vi "Configure.vi"(8 "error in (no error)":errorcluster caption="错误输入（无错误）", 11 "5720A 输入":refnum<class "5720A.lvclass">) -> (0 "error out":errorcluster caption="错误输出", 3 "5720A 输出":refnum<class "5720A.lvclass">)   [LabVIEW 2020, in "5720A.lvlib" / "5720A.lvclass"]
uses:
  5720A.lvclass
  <instrlib>/Fluke 5XXX Series Multicalibrators/Fluke 5XXX Series Multicalibrators.lvlib
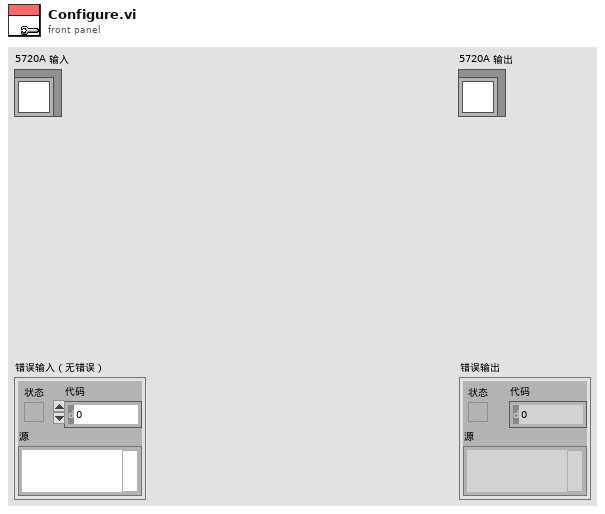
[diagram p1: front panel]
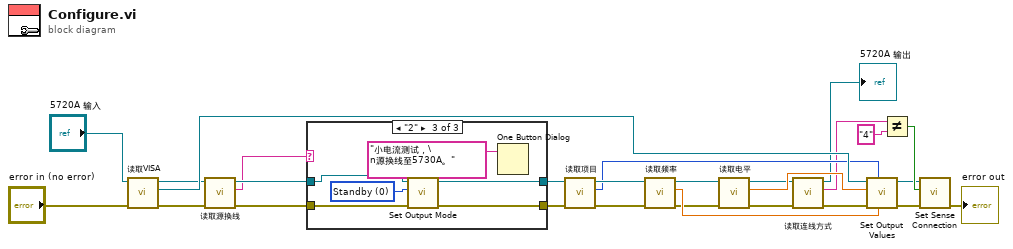
[diagram p0: block diagram]
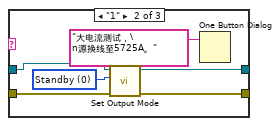
[diagram p3: hidden frame]
diagram:
  n1 = call "读取VISA.vi"("error in (no error)"="error in (no error)", "多功能校准源接口输入"="5720A 输入") -> ("error out"=w6:errorcluster, "VISA"=w26:refnum<visa-resource-name>, "多功能校准源接口输出"=w7:refnum<class "5720A.lvclass">)  [unwired: 7 in]
  n2 = call "读取源换线.vi"("error in (no error)"=w6, "多功能校准源接口输入"=w7) -> ("error out"=w3:errorcluster, "源换线"=w1:string, "多功能校准源接口输出"=w5:refnum<class "5720A.lvclass">)  [unwired: 7 in]
  n3 = case shown="\"2\"" w1 {
    tunnel: w5 -> [w29 w35 w41]
    tunnel: [w29 w32 w38] -> w4
    tunnel: w3 -> [w28 w31 w37]
    tunnel: [w28 w30 w36] -> w2
    frame "0", Default {
    }
    frame "1" {
      w34 = u32 0 items=["Standby", "Operate"] ("Output Mode")
      n4 = call-dynamic "Set Output Mode.vi"("error in (no error)"=w31, "Output Mode"=w34, "5720A 输入"=w35) -> ("error out"=w30:errorcluster, "5720A 输出"=w32:refnum<class "5720A.lvclass">)  [unwired: 7 in]
      n5 = One Button Dialog(message="大电流测试，\n源换线至5725A。" ("消息")) -> ()  [unwired: 1 in, 1 out]
    }
    frame "2" {
      w40 = u32 0 items=["Standby", "Operate"] ("Output Mode")
      n6 = call-dynamic "Set Output Mode.vi"("error in (no error)"=w37, "Output Mode"=w40, "5720A 输入"=w41) -> ("error out"=w36:errorcluster, "5720A 输出"=w38:refnum<class "5720A.lvclass">)  [unwired: 7 in]
      n7 = One Button Dialog(message="小电流测试，\n源换线至5730A。" ("消息")) -> ()  [unwired: 1 in, 1 out]
    }
  }
  n8 = call "读取项目.vi"("error in (no error)"=w2, "多功能校准源接口输入"=w4) -> ("error out"=w22:errorcluster, "项目"=w16:u32, "多功能校准源接口输出"=w19:refnum<class "5720A.lvclass">)  [unwired: 7 in]
  n9 = call "读取频率.vi"("error in (no error)"=w22, "多功能校准源接口输入"=w19) -> ("error out"=w21:errorcluster, "频率"=w25:dbl, "多功能校准源接口输出"=w20:refnum<class "5720A.lvclass">)  [unwired: 7 in]
  n10 = call "读取电平.vi"("error in (no error)"=w21, "多功能校准源接口输入"=w20) -> ("error out"=w14:errorcluster, "电平"=w24:dbl, "多功能校准源接口输出"=w15:refnum<class "5720A.lvclass">)  [unwired: 7 in]
  n11 = call "读取连线方式.vi"("error in (no error)"=w14, "多功能校准源接口输入"=w15) -> ("error out"=w13:errorcluster, "连线方式"=w10:string, "多功能校准源接口输出"=→"5720A 输出":refnum<class "5720A.lvclass">)  [unwired: 7 in]
  n12 = call <instrlib>:"Set Output Values.vi"("Fundamental Frequency (0.0 Hz)"=w25, "Output Value(s) (0 - Amplitude)"=w16, "error in (no error)"=w13, "Primary Value (0.0)"=w24, "VISA resource name"=w26) -> ("error out"=w18:errorcluster, "VISA resource name out"=w8:refnum<visa-resource-name>)  [unwired: 5 in]
  n13 = Not Equal?(x=w10, y="4") -> (x != y?=w9:bool)
  n14 = call <instrlib>:"Set Sense Connection.vi"("error in (no error)"=w18, "Sense Connection (T: Internal)"=w9, "VISA resource name"=w8) -> ("error out"=→"error out":errorcluster)  [unwired: 7 in, 1 out]
